vi "Equate Inputs.vi"(9 "Msg":refnum<class "Msg.lvclass">, 10 "Msg":refnum<class "Msg.lvclass">) -> (2 "Equal":bool)   [LabVIEW 2020, in "jettl.lvlib" / "Msg Specific.lvlib"]
uses:
  Msg/Msg.lvclass
  Msg Specific.lvlib
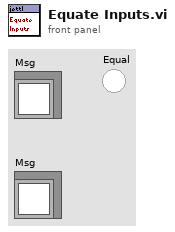
[diagram p1: front panel]
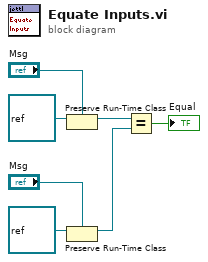
[diagram p0: block diagram]
diagram:
  n1 = Preserve Run-Time Class(object in=refnum<class> refnum ("LabVIEW Object"), 2:"Msg") -> (object out=w3:refnum<class "Msg.lvclass">)  [unwired: 1 in, 1 out]
  n2 = Preserve Run-Time Class(object in=refnum<class> refnum ("LabVIEW Object"), 2:"Msg") -> (object out=w2:refnum<class "Msg.lvclass">)  [unwired: 1 in, 1 out]
  n3 = Equal?(x=w3, y=w2) -> (x = y?=→"Equal":bool)
